vi "addLineToVolume.vi"(5 "tracking":bool, 6 "current volume":T2, 7 "line":T1, 9 "xyz order":bool, 10 "dwellTimeCounter":u32[](array[numeric]), 11 "volume buffer":u32[](array[numeric])) -> (2 "dwellTimeCounter out":u32[](array[numeric]), 3 "volume buffer out":u32[](array[numeric]))   [LabVIEW 2010]
uses:
  volume_info.ctl
  line_info.ctl
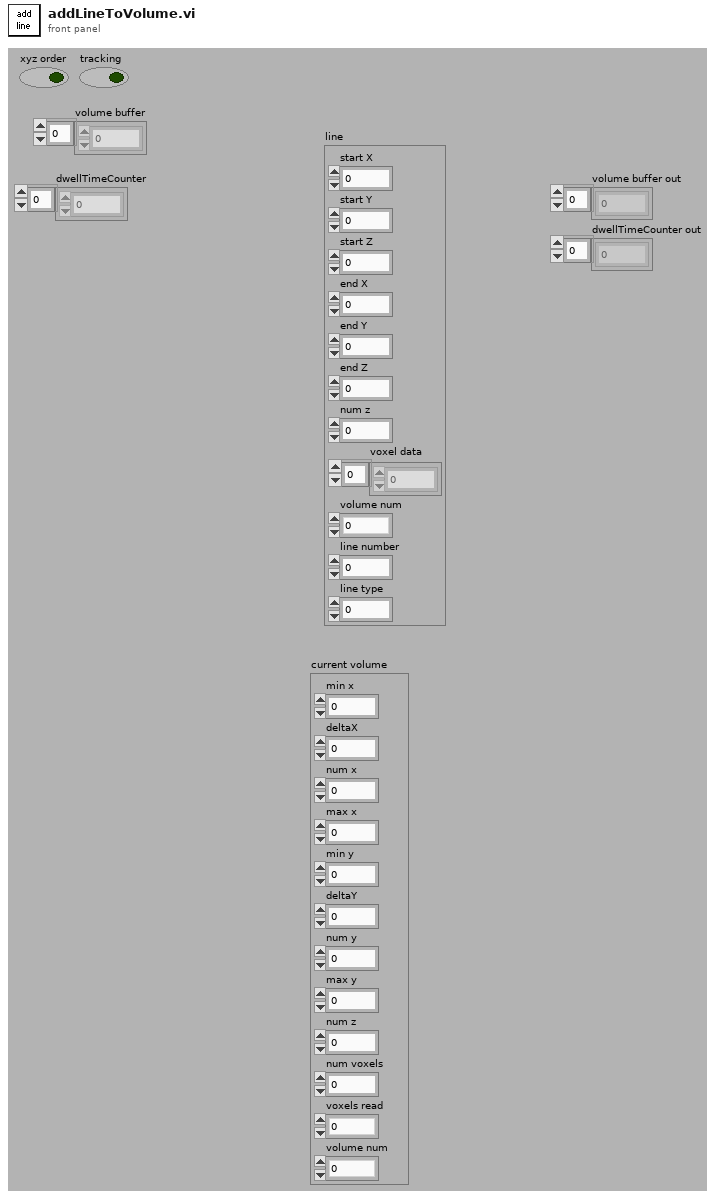
[diagram p1: front panel]
types:
  T1 = typedef "line_info.ctl" = cluster{"start X":i16, "start Y":i16, "start Z":i16, "end X":i16, "end Y":i16, "end Z":i16, "num z":u8, "voxel data":u32[], "volume num":u32, "line number":u16, "line type":u16}
  T2 = typedef "volume_info.ctl" = cluster{"min x":i16, "deltaX":dbl, "num x":u32, "max x":i16, "min y":i16, "deltaY":dbl, "num y":u32, "max y":i16, "num z":u32, "num voxels":u32, "voxels read":u32, "volume num":u32}
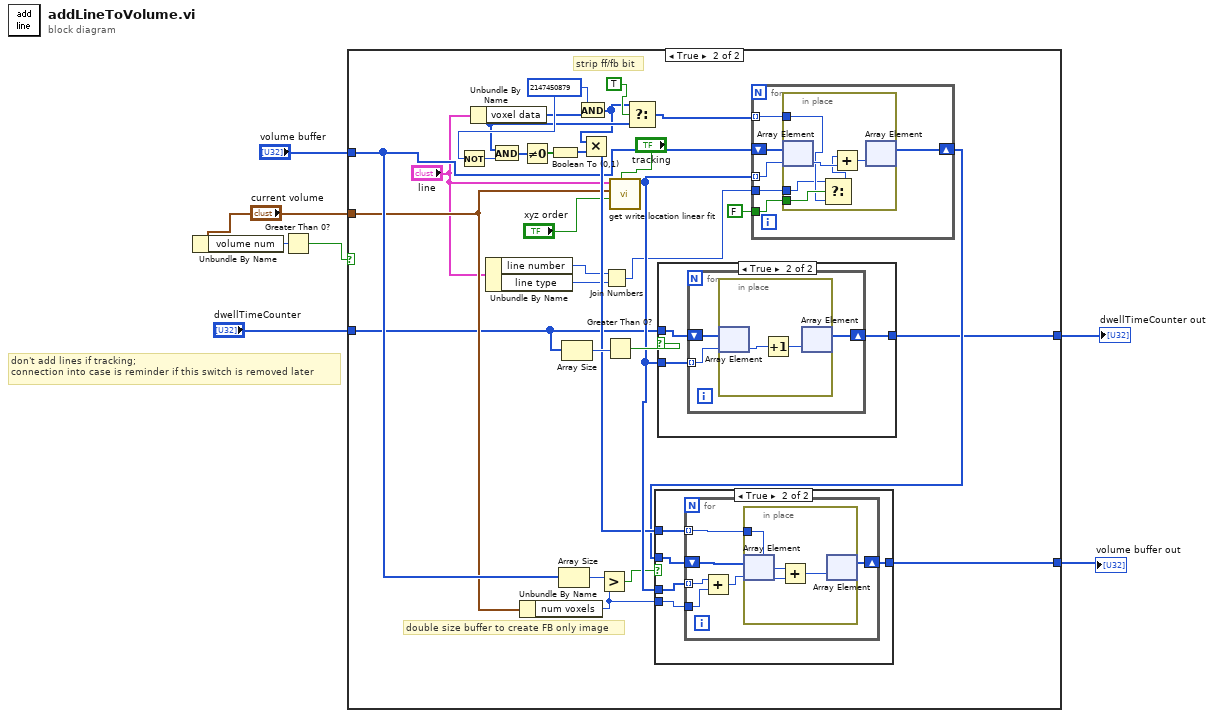
[diagram p0: block diagram]
diagram:
  # "don't add lines if tracking;\nconnection into case is reminder if this switch is removed later"
  n1 = Unbundle By Name("current volume") -> ("volume num"=w5:u32)
  n2 = Greater Than 0?(x=w5) -> (x > 0?=w1:bool)
  n3 = case shown="True" w1 {
    tunnel: "volume buffer" -> [w8 w21]
    tunnel: "current volume" -> [_ w20]
    tunnel: "dwellTimeCounter" -> [w9 w19]
    tunnel: [w9 w18] -> w3
    tunnel: [w8 w17] -> w2
    frame False {
    }
    frame True {
      w33 = u32 2147450879
      # "double size buffer to create FB only image"
      # "strip ff/fb bit"
      n4 = Not(x=w33) -> (.not. x?=w34:u32)
      n5 = Unbundle By Name("line") -> ("voxel data"=w29:u32[])
      n6 = Unbundle By Name("line") -> ("line number"=w15:u16, "line type"=w14:u16)
      n7 = And(x=w29, y=w34) -> (x .and. y?=w32:u32[])
      n8 = Unbundle By Name(w20) -> ("num voxels"=w22:u32)
      n9 = Not Equal To 0?(x=w32) -> (x != 0?=w31:bool[])
      n10 = Boolean To (0,1)(Boolean=w31) -> (0, 1=w30:i16[])
      n11 = Array Size(array=w21) -> (size(s)=w25:i32)
      n12 = Array Size(array=w19) -> (size(s)=w37:i32)
      n13 = And(x=w33, y=w29) -> (x .and. y?=w28:u32[])
      n14 = Multiply(x=w28, y=w30) -> (x*y=w26:u32[])
      n15 = Greater?(x=w25, y=w22) -> (0:w24:bool)
      n16 = Join Numbers(hi=w15, lo=w14) -> ((hi.lo)=w13:u32)
      n17 = Greater Than 0?(x=w37) -> (x > 0?=w38:bool)
      n18 = call "get write location linear fit.vi"("tracking"="tracking", "xyz order"="xyz order", "current volume"=w20, "line"="line") -> ("3D write locations"=w27:u32[])  [unwired: 7 in]
      n19 = Select(t=w28, s=TRUE, f=w29) -> (s? t:f=w36:u32[])
      n20 = case shown="True" w38 {
        tunnel: w19 -> [w54 w57]
        tunnel: [w54 w56] -> w18
        tunnel: w27 -> [_ w55]
        frame False {
        }
        frame True {
          n21 = for {
            tunnel: w55 -> [w59] mode=indexing
            shift-right: [w58] -> w56
            shift-left: w57 -> [w60]
            n22 = in-place {
              n23 = in-place-array #1(w60, w59) -> (w62:u32)
              n24 = Increment(x=w62) -> (x+1=w61:u32)
              n25 = in-place-array #1(w61) -> (w58:u32[])  [unwired: 1 out]
            }
          }
        }
      }
      n26 = for {
        tunnel: w27 -> [w66] mode=indexing
        tunnel: w36 -> [w68] mode=indexing
        shift-right: [w65] -> w23
        shift-left: w21 -> [w67]
        tunnel: w13 -> [w64]
        tunnel: FALSE ("use line and frame numbers") -> [w63]
        n27 = in-place {
          in-place-border: w68 -> [w71]
          in-place-border: w64 -> [w70]
          in-place-border: w63 -> [w72]
          n28 = in-place-array #2(w67, w66) -> (w74:u32)
          n29 = Select(t=w70, s=w72, f=w71) -> (s? t:f=w69:u32)
          n30 = Add(x=w69, y=w74) -> (x+y=w73:u32)
          n31 = in-place-array #2(w73) -> (w65:u32[])  [unwired: 1 out]
        }
      }
      n32 = case shown="True" w24 {
        tunnel: w23 -> [w39 w44]
        tunnel: [w39 w43] -> w17
        tunnel: w27 -> [_ w42]
        tunnel: w26 -> [_ w41]
        tunnel: w22 -> [_ w40]
        frame False {
        }
        frame True {
          n33 = for {
            tunnel: w42 -> [w46] mode=indexing
            shift-right: [w49] -> w43
            shift-left: w44 -> [w50]
            tunnel: w41 -> [w48] mode=indexing
            tunnel: w40 -> [w45]
            n34 = Add(x=w46, y=w45) -> (x+y=w47:u32)
            n35 = in-place {
              in-place-border: w48 -> [w53]
              n36 = in-place-array #3(w50, w47) -> (w52:u32)
              n37 = Add(x=w53, y=w52) -> (x+y=w51:u32)
              n38 = in-place-array #3(w51) -> (w49:u32[])  [unwired: 1 out]
            }
          }
        }
      }
    }
  }
  "dwellTimeCounter out" <- w3
  "volume buffer out" <- w2
